vi "Convert B_ID to D_ID.vi"(1 "Opt H?":bool, 2 "Opt F?":bool, 3 "Opt. D?":bool, 7 "B-series ID":i32) -> (8 "Config 'D' ID":u32)   [LabVIEW 2011]
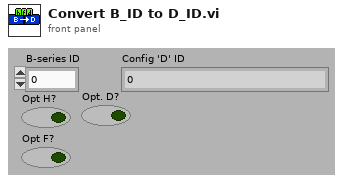
[diagram p1: front panel]
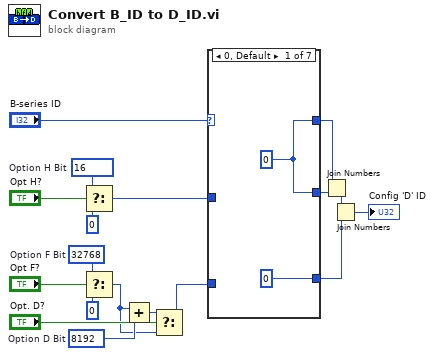
[diagram p0: block diagram]
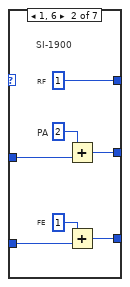
[diagram p2: hidden frame]
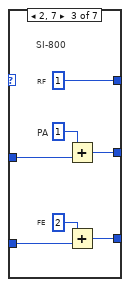
[diagram p3: hidden frame]
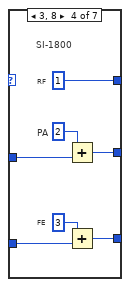
[diagram p4: hidden frame]
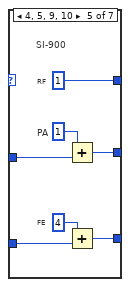
[diagram p5: hidden frame]
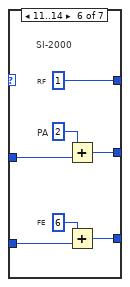
[diagram p6: hidden frame]
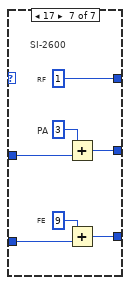
[diagram p7: hidden frame]
diagram:
  w5 = u16 8192  # Option D Bit
  w12 = u16 32768  # Option F Bit
  w17 = u8 16  # Option H Bit
  n1 = Select(t=w17, s="Opt H?", f=u8 0) -> (s? t:f=w14:u8)
  n2 = Select(t=w12, s="Opt F?", f=u16 0) -> (s? t:f=w2:u16)
  n3 = Add(x=w2, y=w5) -> (x+y=w3:u16)
  n4 = Select(t=w3, s="Opt. D?", f=w2) -> (s? t:f=w1:u16)
  n5 = case shown="0, Default" "B-series ID" {
    tunnel: w14 -> [_ w26 w33 w40 w47 w54 w58]
    tunnel: w1 -> [_ w27 w34 w41 w48 w55 w57]
    tunnel: [w20 u8 1 ("RF") u8 1 ("RF") u8 1 ("RF") u8 1 ("RF") u8 1 ("RF") u8 1 ("RF")] -> w7
    tunnel: [w20 w22 w29 w36 w43 w50 w59] -> w8
    tunnel: [u16 0 ("FE") w21 w28 w35 w42 w49 w56] -> w9
    frame 0, Default {
      w20 = u8 0
    }
    frame 1, 6 {
      # "FE"
      # "PA"
      # "RF"
      # "SI-1900"
      n6 = Add(x=u8 2 ("RF"), y=w26) -> (x+y=w22:u8)
      n7 = Add(x=u16 1 ("FE"), y=w27) -> (x+y=w21:u16)
    }
    frame 2, 7 {
      # "FE"
      # "PA"
      # "RF"
      # "SI-800"
      n8 = Add(x=u8 1 ("RF"), y=w33) -> (x+y=w29:u8)
      n9 = Add(x=u16 2 ("FE"), y=w34) -> (x+y=w28:u16)
    }
    frame 3, 8 {
      # "FE"
      # "PA"
      # "RF"
      # "SI-1800"
      n10 = Add(x=u8 2 ("RF"), y=w40) -> (x+y=w36:u8)
      n11 = Add(x=u16 3 ("FE"), y=w41) -> (x+y=w35:u16)
    }
    frame 4, 5, 9, 10 {
      # "FE"
      # "PA"
      # "RF"
      # "SI-900"
      n12 = Add(x=u8 1 ("RF"), y=w47) -> (x+y=w43:u8)
      n13 = Add(x=u16 4 ("FE"), y=w48) -> (x+y=w42:u16)
    }
    frame 11..14 {
      # "FE"
      # "PA"
      # "RF"
      # "SI-2000"
      n14 = Add(x=u8 2 ("RF"), y=w54) -> (x+y=w50:u8)
      n15 = Add(x=u16 6 ("FE"), y=w55) -> (x+y=w49:u16)
    }
    frame 17 {
      # "FE"
      # "PA"
      # "RF"
      # "SI-2600"
      n16 = Add(x=u8 3 ("RF"), y=w58) -> (x+y=w59:u8)
      n17 = Add(x=u16 9 ("FE"), y=w57) -> (x+y=w56:u16)
    }
  }
  n18 = Join Numbers(hi=w7, lo=w8) -> ((hi.lo)=w10:u16)
  n19 = Join Numbers(hi=w10, lo=w9) -> ((hi.lo)=→"Config 'D' ID":u32)
